vi "append_status_updates_to_results.vi"(4 "part_ID":string, 6 "operation_ID":string, 7 "opeartion_status":u8, 8 "error_in":errorcluster, 11 "INSERT_statements":string[](array[string])) -> (0 "error_out":errorcluster, 3 "INSERT_statements_with_status_updates":string[](array[string]))   [LabVIEW 2020]
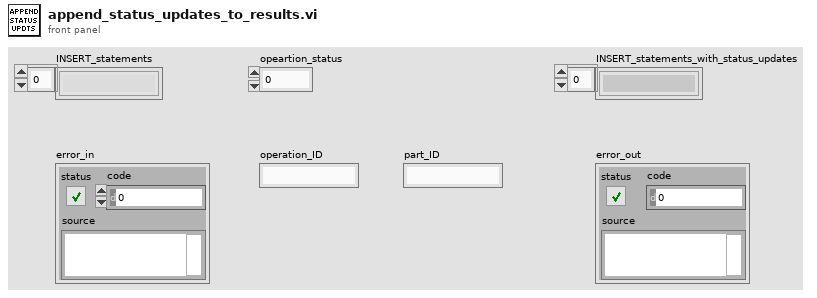
[diagram p1: front panel]
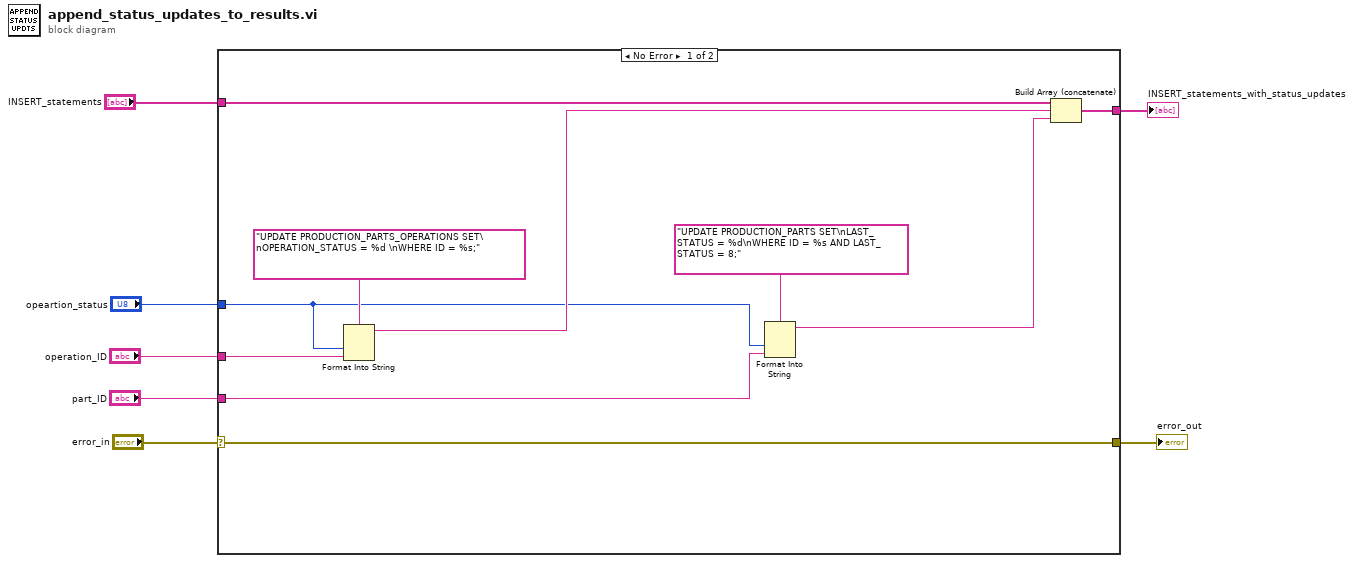
[diagram p0: block diagram]
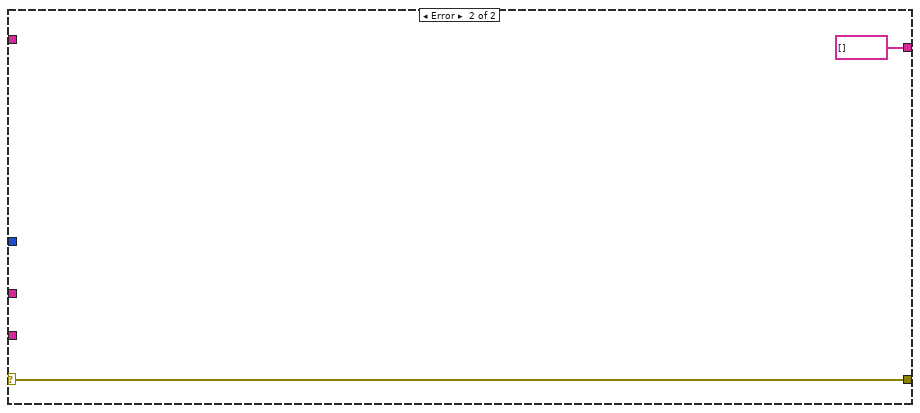
[diagram p2: hidden frame]
diagram:
  n1 = case shown="No Error" "error_in" {
    selector: "error_in" -> [w12 w19]
    tunnel: "INSERT_statements" -> [w16 _]
    tunnel: [w13 string[] [] ("INSERT_statements")] -> w6
    tunnel: "operation_ID" -> [w17 _]
    tunnel: [w12 w19] -> w3
    tunnel: "part_ID" -> [w11 _]
    tunnel: "opeartion_status" -> [w8 _]
    frame No Error {
      n2 = Format Into String(format string="UPDATE PRODUCTION_PARTS_OPERATIONS SET\nOPERATION_STATUS = %d \nWHERE ID = %s;", w8, w17) -> (resulting string=w14:string)  [unwired: 2 in, 1 out]
      n3 = Format Into String(format string="UPDATE PRODUCTION_PARTS SET\nLAST_STATUS = %d\nWHERE ID = %s AND LAST_STATUS = 8;", w8, w11) -> (resulting string=w9:string)  [unwired: 2 in, 1 out]
      n4 = Build Array (concatenate)(w16, w14, w9) -> (w13:string[])
    }
    frame Error {
    }
  }
  "INSERT_statements_with_status_updates" <- w6
  "error_out" <- w3
